vi "StandardEngineUI.vi"() -> ()   [LabVIEW 2013, in "Standard Engine Editor Node.lvclass"]
doc: "This VI is a template of the minimun components for a node UI.\nIt shows how to use the queue and the user event."
uses:
  Standard Engine Editor Node.lvclass
  <vilib>/CEF_TreeControl/Node/NodeRef.ctl
  <vilib>/CEF_TreeControl/Node/NISE_CEF_Node.lvclass
  <vilib>/NI/AMC/Message Queue.ctl
  <vilib>/NI/AMC/Message.ctl
  <vilib>/NI/Tools/Keyed Array/KeyedArray.ctl
  <vilib>/CEF_TreeControl/Node/UserEventRef.ctl
  <vilib>/CEF_TreeControl/Controls/EventCluster.ctl
  <vilib>/NI/TBM Engines/Standard Engine/Configuration/Supported Timing Sources.ctl
  Processor Assignment Mode.ctl
  <vilib>/NI/TBM Engines/Standard Engine/Configuration/Module Decimation.ctl
  <vilib>/NI/TBM Engines/Standard Engine/Configuration/Standard Engine Configuration.lvclass
  <vilib>/NI/Tag Bus Data Framework/Configuration Editor/Classes/Engine Parent/Engine Parent Editor Node.lvclass
  <vilib>/NI/TBM Engines/Standard Engine/Configuration/Standard Engine Configuration.lvclass/Standard Engine Configuration.ctl
  <vilib>/NI/TBM Engines/Standard Engine/Configuration/Module Error Configuration.ctl
  <vilib>/NI/TBM Engines/Standard Engine/Configuration/Error Actions By Category.ctl
  <vilib>/NI/Tag Bus Module Framework/runtime/error classification.ctl
  <vilib>/NI/TBM Engines/Standard Engine/Configuration/Error Actions.ctl
  <vilib>/NI/TBM Engines/Standard Engine/Configuration/Write Timing Source Type.vi
  <vilib>/NI/TBM Engines/Standard Engine/Configuration/Write Processor.vi
  <vilib>/NI/TBM Engines/Standard Engine/Configuration/Read Module Specific Configuration.vi
  <vilib>/NI/TBM Engines/Standard Engine/Configuration/Read Processor.vi
  <vilib>/NI/TBM Engines/Standard Engine/Configuration/Read Timing Source Type.vi
  <vilib>/NI/Tag Bus Data Framework/Configuration Editor/Classes/Engine Parent/Read Name.vi
  <vilib>/NI/AMC/Create Single Message.vi
  <vilib>/NI/AMC/Update Message Routing Info.vi
  <vilib>/NI/Tag Bus Module Framework/root configuration/read metadata property.vi
  <vilib>/NI/TBM Engines/Standard Engine/Configuration/Write Timing Source dt.vi
  <vilib>/NI/AMC/Send Message.vi
  <vilib>/NI/TBM Engines/Standard Engine/Configuration/Read Timing Source dt.vi
  <vilib>/NI/TBM Engines/Standard Engine/Configuration/Find Module Specific Config.vi
  <vilib>/Utility/error.llb/Error Cluster From Error Code.vi
  <vilib>/NI/Tag Bus Module Framework/root configuration/TBM configuration.lvclass
  <vilib>/NI/AMC/AMC.lvlib
  <vilib>/NI/Tag Bus Module Framework/runtime/TBM module execution interface.lvclass
  <vilib>/CEF_TreeControl/NISE_CEF_TreeControl.lvlib
  <vilib>/NI/Tools/Keyed Array/Tools_KeyedArray.lvlib
panel:
  in  "Warning Message":string="This timing source is not deterministic."
  in  "Module Decimation":T2(array[cluster]) {"Module Decimation"."Decimation" min=1}
  in  "Mode":T3
  in  "Timing Source Type":T4=enum."1 kHz Clock"
  in  "Engine Name":string
  in  "Procesor Assignment":i32 min=0
  in  "Timing Source dt":u32=5000
  in  "user event":T5
  in  "main queue":T6
  in  "node ref":T7
  # "Processor Assignment"
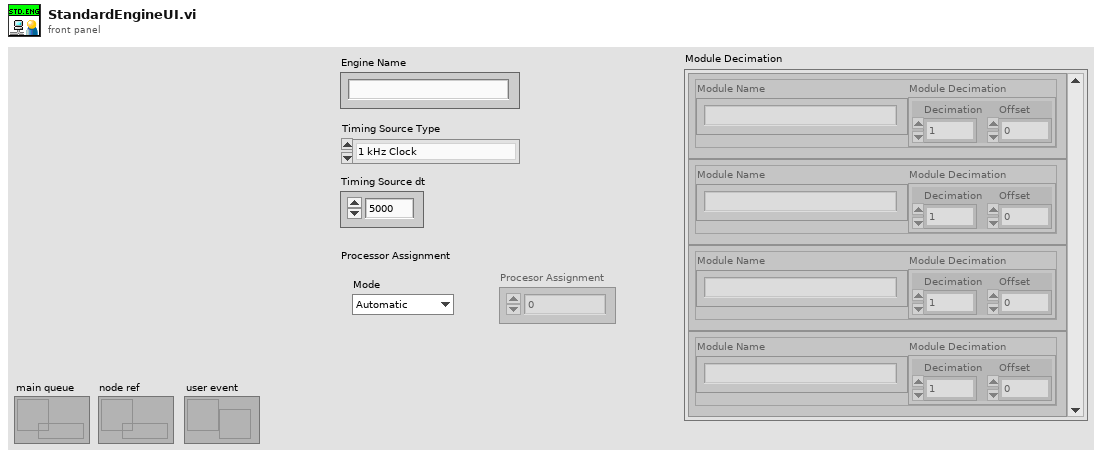
[diagram p1: front panel]
types:
  T1 = typedef "Standard Engine Configuration.lvclass/Module Decimation.ctl" = cluster{"Decimation":u16, "Offset":u16}
  T2 = cluster{"Module Name":string, "Module Decimation":T1, "Module ID":string}[]
  T3 = typedef "Standard Engine Editor Node.lvclass/Processor Assignment Mode.ctl" = enum16{"Automatic", "Manual"}
  T4 = typedef "Standard Engine Configuration.lvclass/Supported Timing Sources.ctl" = enum16{"Use Module Timing Source", "1 kHz Clock", "1 MHz Clock", "Synchronize to Scan Engine"}
  T5 = typedef "NISE_CEF_Node.lvclass/UserEventRef.ctl" = refnum<user-event>
  T6 = typedef "AMC.lvlib/Message Queue.ctl" = refnum<queue>
  T7 = typedef "NISE_CEF_Node.lvclass/NodeRef.ctl" = refnum<data-value>
  T8 = typedef "NISE_CEF_TreeControl.lvlib/EventCluster.ctl" = cluster{"command":string, "data":string}
  T9 = typedef "Standard Engine Configuration.lvclass/Module Error Configuration.ctl" = cluster{"Module Error Configuration":T10[]}
  T10 = typedef "Standard Engine Configuration.lvclass/Error Actions By Category.ctl" = cluster{"error classification":T11, "Error Actions":T12[]}
  T11 = typedef "TBM module execution interface.lvclass/error classification.ctl" = enum16{"unknown", "none", "trivial", "recoverable", "critical"}
  T12 = typedef "Standard Engine Configuration.lvclass/Error Actions.ctl" = enum16{"Clear", "Notify", "Stop Component", "Stop Engine", "Safe State", "Attempt Recovery"}
  T13 = typedef "Standard Engine Configuration.lvclass/Module Specific Configuration.ctl" = cluster{"Module ID":string, "Module Decimation":T1, "Module Error Configuration":T9}
  T14 = cluster{"Module Name":string, "Module Decimation":T1, "Module ID":string}
  T15 = enum8{"Enabled", "Disabled", "Disabled and Grayed Out"}
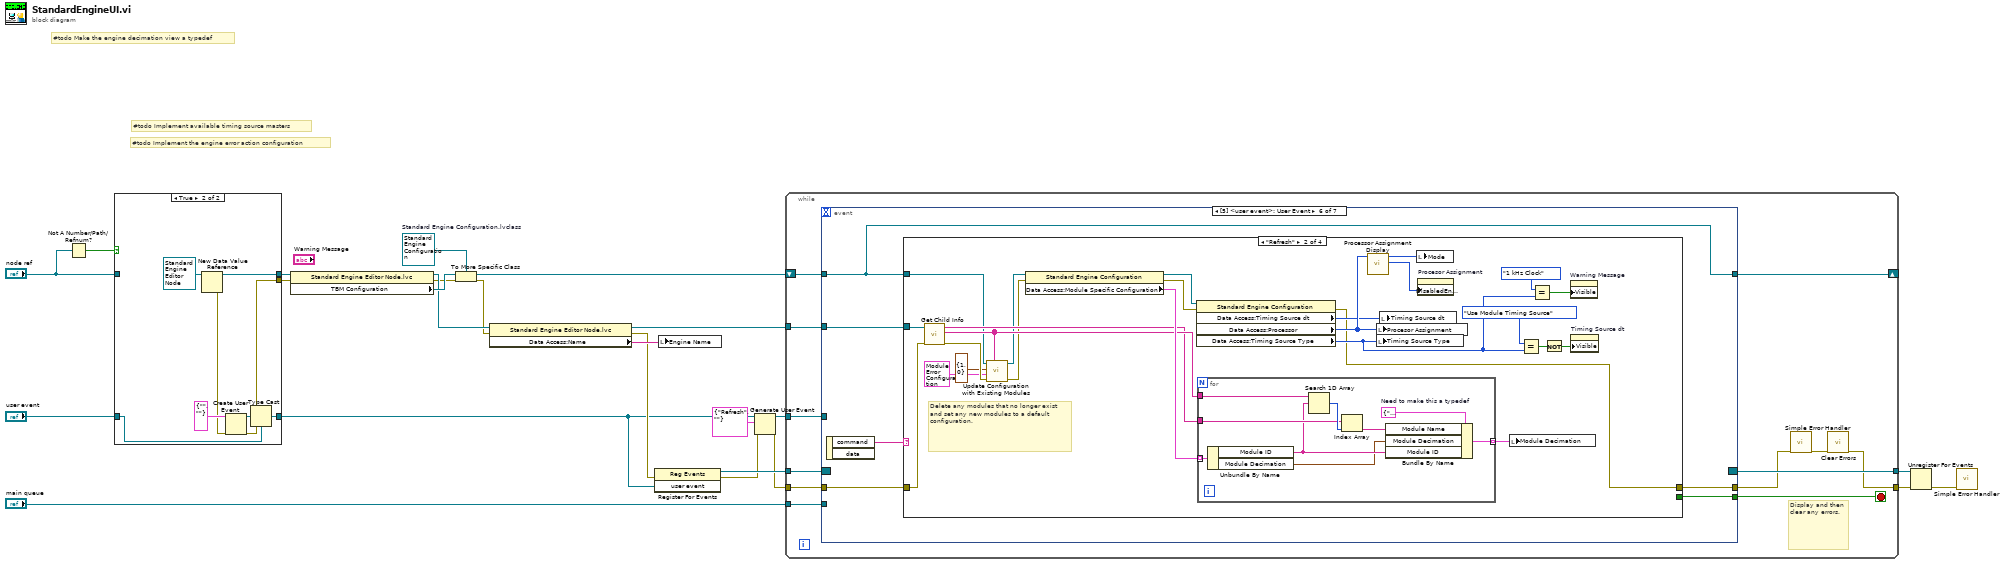
[diagram p0: block diagram]
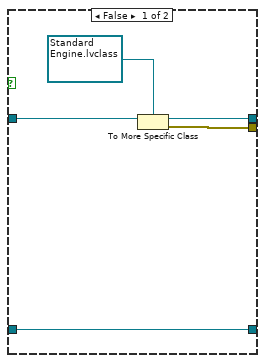
[diagram p2: hidden frame]
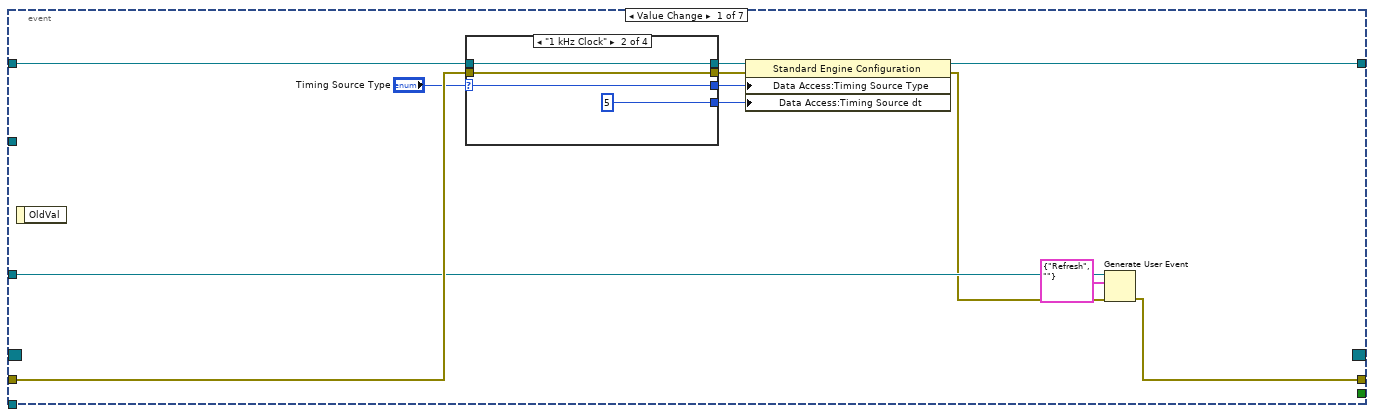
[diagram p3: hidden frame]
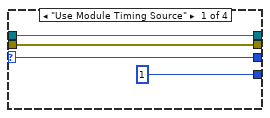
[diagram p4: hidden frame]
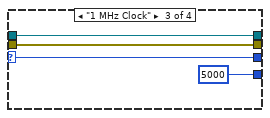
[diagram p5: hidden frame]
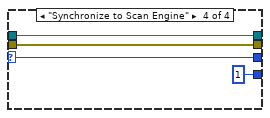
[diagram p6: hidden frame]
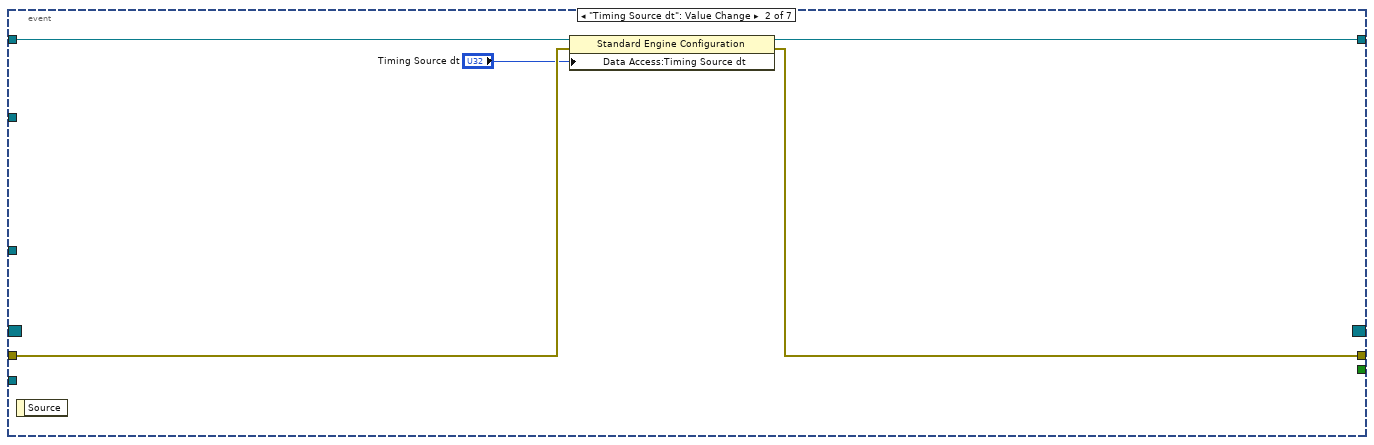
[diagram p7: hidden frame]
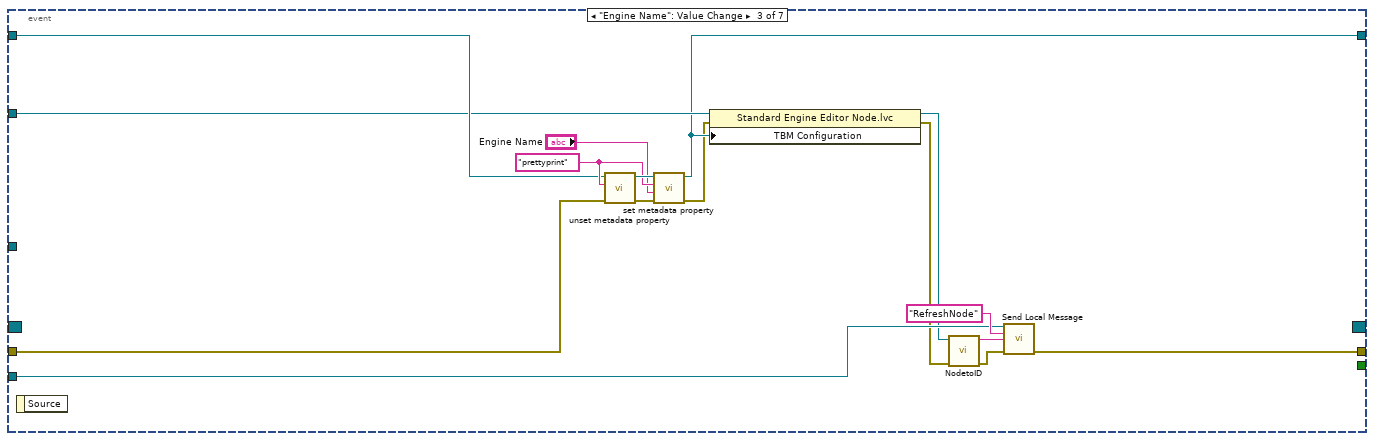
[diagram p8: hidden frame]
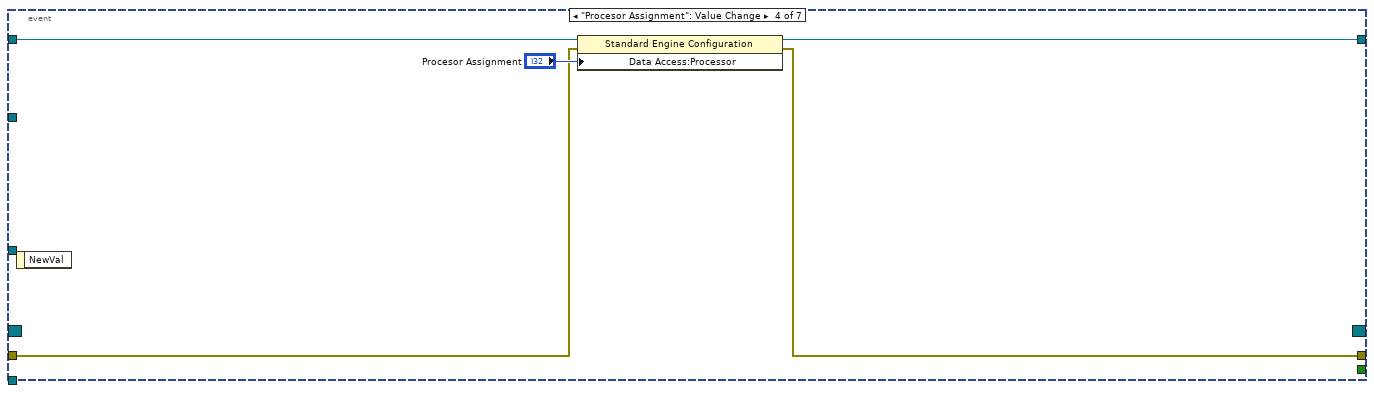
[diagram p9: hidden frame]
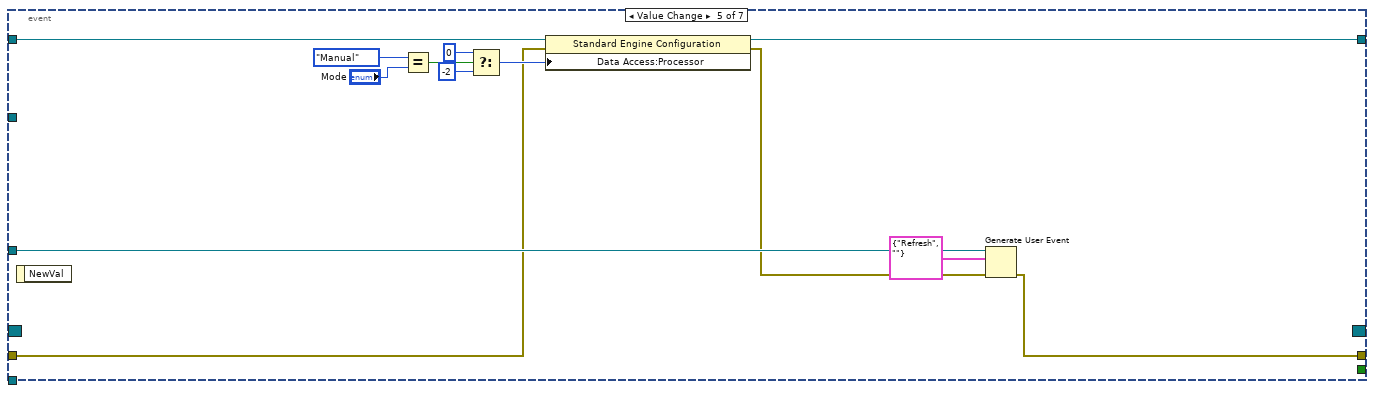
[diagram p10: hidden frame]
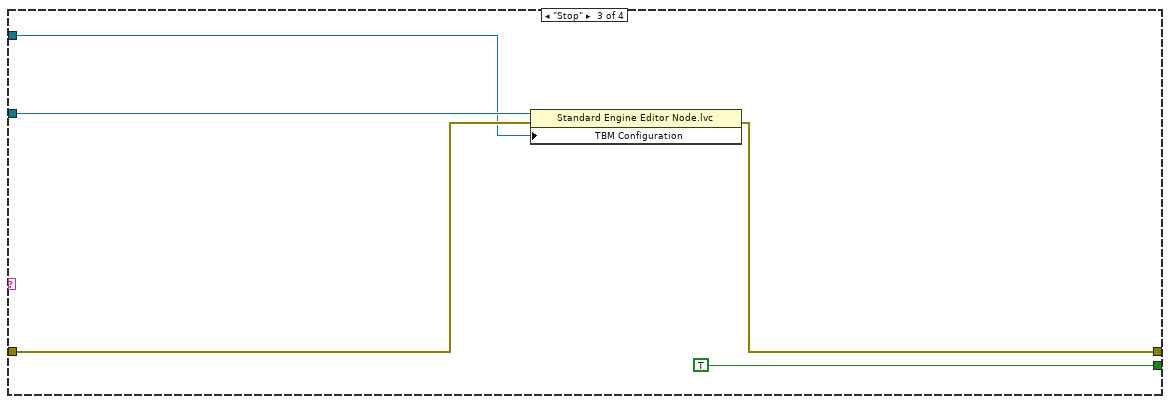
[diagram p12: hidden frame]
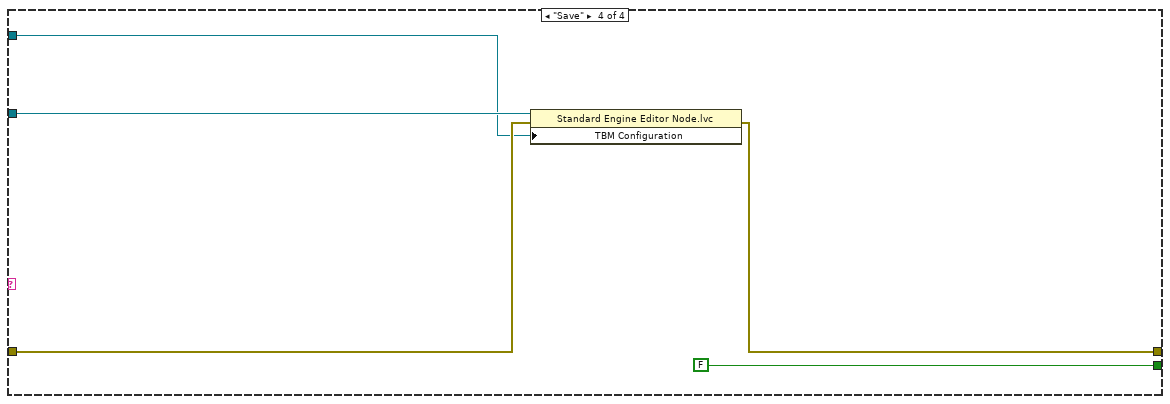
[diagram p13: hidden frame]
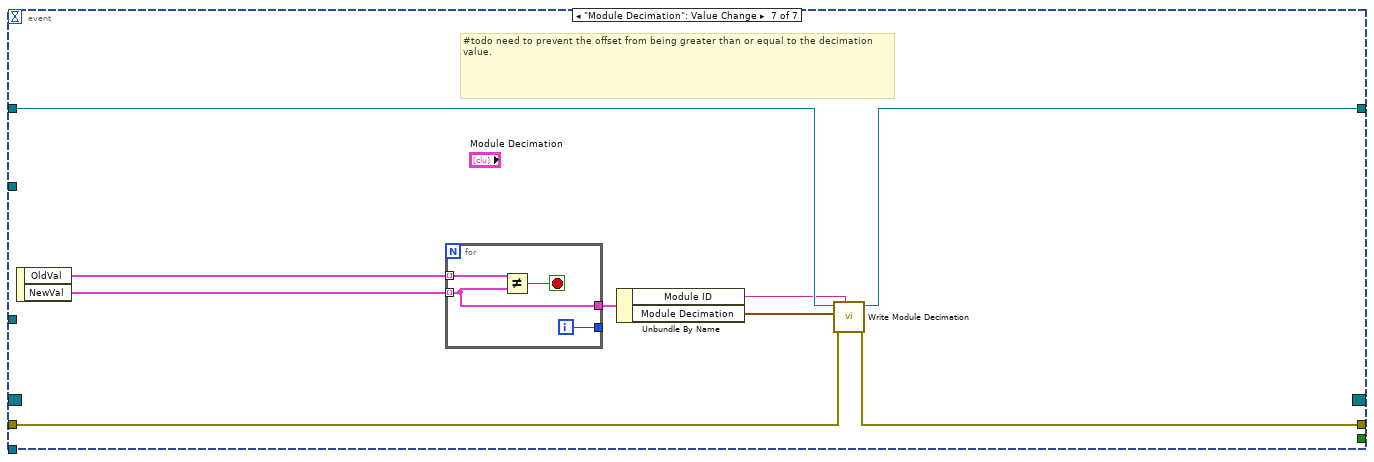
[diagram p14: hidden frame]
diagram:
  w20 = refnum<class "Standard Engine Configuration.lvclass"> refnum  # Standard Engine Configuration.lvclass
  # "#todo Implement the engine error action configuration"
  # "#todo Implement available timing source masters"
  # "#todo Make the engine decimation view a typedef"
  n1 = Not A Number/Path/Refnum?(number/path/refnum="node ref") -> (NaN/Path/Refnum?=w11:bool)
  n2 = case shown="True" w11 {
    tunnel: [w28 w32] -> w10
    tunnel: [w27 w36] -> w18
    tunnel: "node ref" -> [w26 _]
    tunnel: "user event" -> [w25 w30]
    tunnel: [w25 w31] -> w1
    frame False {
      n3 = To More Specific Class(target class=refnum<data-value> refnum ("data value reference"), reference=w26) -> (specific class reference=w27:refnum<data-value>, error out=w28:errorcluster)  [unwired: 1 in]
    }
    frame True {
      n4 = New Data Value Reference(data value=refnum<class "Standard Engine Editor Node.lvclass"> refnum ("Standard Engine Editor Node.lvclass")) -> (data value reference=w36:refnum<data-value>, error out=w33:errorcluster)  [unwired: 1 in]
      n5 = Create User Event(user event datatype=T8 {"command"="", "data"=""} ("event data"), error in=w33) -> (user event=w34:refnum<user-event>, error out=w32:errorcluster)
      n6 = Type Cast(type=w30, x=w34) -> (*(type *) &x=w31:T5)
    }
  }
  n7 = property class="Standard Engine Editor Node.lvc"(reference=w18, error in=w10) -> (reference out=w16:refnum<data-value>, error out=w15:errorcluster, "TBM Configuration"=w17:refnum<class "TBM configuration.lvclass">)
  n8 = To More Specific Class(target class=w20, reference=w17, error in=w15) -> (specific class reference=w8:refnum<class "Standard Engine Configuration.lvclass">, error out=w13:errorcluster)
  n9 = property class="Standard Engine Editor Node.lvc"(reference=w16, error in=w13) -> (reference out=w9:refnum<data-value>, error out=w7:errorcluster, "Data Access:Name"=w19:string)
  n10 = register-events(error in=w7, w1) -> (reference out=w23:refnum<event-registration>, error out=w6:errorcluster)  [unwired: 1 in]
  n11 = local write "Engine Name"(w19) -> ()
  n12 = Generate User Event(user event=w1, event data cluster=T8 {"command"="Refresh", "data"=""} ("event data"), error in=w6) -> (user event out=w3:T5, error out=w5:errorcluster)  [unwired: 1 in]
  n13 = while {
    tunnel: "main queue" -> [w49]
    tunnel: w23 -> [w48]
    tunnel: [w47] -> w22
    tunnel: [w40] -> w21
    tunnel: w5 -> [w45]
    shift-right: [w44] -> _
    shift-left: w8 -> [w39]
    tunnel: w9 -> [w43]
    tunnel: w3 -> [w38]
    stop <- w46 stop-if-true
    # "Display and then clear any errors."
    n14 = event shown="[5] <user event>: User Event" {
      selector: w48 -> [_ _ _ _ _ _ _]
      dyn-events: [_ _ _ _ _ _ _] -> w47
      timeout: _ -> [_ _ _ _ _ _ _]
      tunnel: w49 -> [_ _ w97 _ _ _ _]
      tunnel: [_ _ _ _ _ w122 _] -> w46
      tunnel: [w51 w79 w95 w99 w105 w119 w170] -> w42
      tunnel: w45 -> [w58 w80 w90 w100 w104 w120 w171]
      tunnel: w39 -> [w60 w82 w89 w103 w116 w117 w174]
      tunnel: [w61 w81 w86 w102 w115 w117 w173] -> w44
      tunnel: w43 -> [_ _ w87 _ _ w121 _]
      tunnel: w38 -> [w53 _ _ _ w107 _ _]
      event Value Change {
        n15 = event-data() -> ()  [unwired: 1 in, 1 out]
        n16 = case shown="\"1 kHz Clock\"" "Timing Source Type" {
          selector: "Timing Source Type" -> [w65 w69 w71 w75]
          tunnel: w60 -> [w64 w68 w73 w77]
          tunnel: [w64 w68 w73 w77] -> w59
          tunnel: w58 -> [w63 w67 w72 w76]
          tunnel: [w63 w67 w72 w76] -> w57
          tunnel: [w65 w69 w71 w75] -> w50
          tunnel: [u32 1 ("Timing Source dt") u32 5 ("Timing Source dt") u32 5000 ("Timing Source dt") u32 1 ("Timing Source dt")] -> w55
          frame "Use Module Timing Source" {
          }
          frame "1 kHz Clock" {
          }
          frame "1 MHz Clock" {
          }
          frame "Synchronize to Scan Engine" {
          }
        }
        n17 = property class="Standard Engine Configuration"(reference=w59, error in=w57, "Data Access:Timing Source Type"=w50, "Data Access:Timing Source dt"=w55) -> (reference out=w61:refnum<class "Standard Engine Configuration.lvclass">, error out=w52:errorcluster)
        n18 = Generate User Event(user event=w53, event data cluster=T8 {"command"="Refresh", "data"=""} ("event data"), error in=w52) -> (error out=w51:errorcluster)  [unwired: 1 in, 1 out]
      }
      event "Timing Source dt": Value Change {
        n19 = event-data() -> ()  [unwired: 1 in, 1 out]
        n20 = property class="Standard Engine Configuration"(reference=w82, error in=w80, "Data Access:Timing Source dt"="Timing Source dt") -> (reference out=w81:refnum<class "Standard Engine Configuration.lvclass">, error out=w79:errorcluster)
      }
      event "Engine Name": Value Change {
        w91 = "prettyprint" ("key")
        n21 = event-data() -> ()  [unwired: 1 in, 1 out]
        n22 = call <vilib>:"unset metadata property.vi"("error in"=w90, "key"=w91, "configuration in"=w89) -> ("error out"=w92:errorcluster, "configuration out"=w93:refnum<class "Standard Engine Configuration.lvclass">)  [unwired: 7 in]
        n23 = call <vilib>:"set metadata property.vi"("error in"=w92, "value"="Engine Name", "key"=w91, "configuration in"=w93) -> ("error out"=w85:errorcluster, "configuration out"=w86:refnum<class "Standard Engine Configuration.lvclass">)  [unwired: 6 in]
        n24 = property class="Standard Engine Editor Node.lvc"(reference=w87, error in=w85, "TBM Configuration"=w86) -> (reference out=w83:refnum<data-value>, error out=w84:errorcluster)
        n25 = call <vilib>:"NodetoID.vi"("error in"=w84, "node ref"=w83) -> ("error out"=w94:errorcluster, "ID"=w96:string)  [unwired: 8 in]
        n26 = call <vilib>:"Send Local Message.vi"("message queue in"=w97, "message name"="RefreshNode" ("Message Name"), "message value"=w96, "error in"=w94) -> ("error out"=w95:errorcluster)  [unwired: 9 in, 2 out]
      }
      event "Procesor Assignment": Value Change {
        n27 = event-data() -> ()  [unwired: 1 in, 1 out]
        n28 = property class="Standard Engine Configuration"(reference=w103, error in=w100, "Data Access:Processor"="Procesor Assignment") -> (reference out=w102:refnum<class "Standard Engine Configuration.lvclass">, error out=w99:errorcluster)
      }
      event Value Change {
        n29 = event-data() -> ()  [unwired: 1 in, 1 out]
        n30 = Equal?(x=Processor_Assignment_Mode."Manual", y="Mode") -> (x = y?=w109:bool)
        n31 = Select(t=0, s=w109, f=-2 ("Processor")) -> (s? t:f=w110:i32)
        n32 = property class="Standard Engine Configuration"(reference=w116, error in=w104, "Data Access:Processor"=w110) -> (reference out=w115:refnum<class "Standard Engine Configuration.lvclass">, error out=w106:errorcluster)
        n33 = Generate User Event(user event=w107, event data cluster=T8 {"command"="Refresh", "data"=""} ("event data"), error in=w106) -> (error out=w105:errorcluster)  [unwired: 1 in, 1 out]
      }
      event User Event {
        n34 = event-data() -> ("command"=w118:string)  [unwired: 1 in, 1 out]
        n35 = case shown="\"Refresh\"" w118 {
          tunnel: [_ _ TRUE FALSE] -> w122
          tunnel: w121 -> [_ w143 w161 w166]
          tunnel: w120 -> [w123 w140 w160 w165]
          tunnel: [w123 w129 w159 w164] -> w119
          tunnel: w117 -> [_ w128 w158 w163]
          frame Default {
          }
          frame "Refresh" {
            # "Delete any modules that no longer exist and set any new modules to a default configuration."
            n36 = call "Get Child Info.vi"("error in (no error)"=w140, "Data Value Reference in"=w143) -> ("error out"=w146:errorcluster, "Instance Identifier"=w142:string[], "Display Names"=w141:string[])  [unwired: 7 in]
            n37 = call <vilib>:"Update Configuration with Existing Modules.vi"("Module IDs"=w142, "error in"=w146, "Default Module Error Configuration"=T9 {"Module Error Configuration"=[{"error classification"=enum."unknown", "Error Actions"=[enum."Stop Engine"]}, {"error classification"=enum."none", "Error Actions"=[enum."Stop Engine"]}, {"error classification"=enum."trivial", "Error Actions"=[enum."Stop Engine"]}, {"error classification"=enum."recoverable", "Error Actions"=[enum."Stop Engine"]}, {"error classification"=enum."critical", "Error Actions"=[enum."Stop Engine"]}]} ("Module Error Configuration"), "Default Module Decimation"=T1 {"Decimation"=1, "Offset"=0}, "Standard Engine Configuration in"=w128) -> ("error out"=w125:errorcluster, "Standard Engine Configuration out"=w127:refnum<class "Standard Engine Configuration.lvclass">)  [unwired: 5 in]
            n38 = property class="Standard Engine Configuration"(reference=w127, error in=w125) -> (reference out=w126:refnum<class "Standard Engine Configuration.lvclass">, error out=w124:errorcluster, "Data Access:Module Specific Configuration"=w147:T13[])
            n39 = property class="Standard Engine Configuration"(reference=w126, error in=w124) -> (error out=w129:errorcluster, "Data Access:Timing Source dt"=w130:u32, "Data Access:Processor"=w131:i32, "Data Access:Timing Source Type"=w136:T4)  [unwired: 1 out]
            n40 = for {
              tunnel: w147 -> [w157] mode=indexing
              tunnel: w142 -> [w156]
              tunnel: w141 -> [w154]
              tunnel: [w149] -> w148 mode=indexing
              w153 = T14 {"Module Name"="", "Module Decimation"={"Decimation"=1, "Offset"=0}, "Module ID"=""}  # Need to make this a typedef
              n41 = Unbundle By Name(w157) -> ("Module ID"=w151:string, "Module Decimation"=w150:T1)
              n42 = Search 1D Array(1D array=w156, element=w151) -> (index of element=w155:i32)  [unwired: 1 in]
              n43 = Index Array(array=w154, index=w155) -> (element=w152:string)
              n44 = Bundle By Name(cluster=w153, "Module Name"=w152, "Module Decimation"=w150, "Module ID"=w151) -> (w149:T14)
            }
            n45 = call "Processor Assignment Display.vi"("Data Access:Processor"=w131) -> ("Enabled?"=w133:T15, "Mode"=w132:T3)  [unwired: 9 in]
            n46 = local write "Procesor Assignment"(w131) -> ()
            n47 = local write "Timing Source Type"(w136) -> ()
            n48 = local write "Timing Source dt"(w130) -> ()
            n49 = local write "Mode"(w132) -> ()
            n50 = property on="Procesor Assignment" class="DigNum (strict)"("DisabledEnum"=w133) -> ()  [unwired: 2 in, 2 out]
            n51 = local write "Module Decimation"(w148) -> ()
            n52 = Equal?(x=Supported_Timing_Sources."Use Module Timing Source" ("Timing Source Type"), y=w136) -> (x = y?=w138:bool)
            n53 = Equal?(x=Supported_Timing_Sources."1 kHz Clock" ("Timing Source Type"), y=w136) -> (x = y?=w134:bool)
            n54 = Not(x=w138) -> (.not. x?=w139:bool)
            n55 = property on="Warning Message" class="Str"("Visible"=w134) -> ()  [unwired: 2 in, 2 out]
            n56 = property on="Timing Source dt" class="DigNum (strict)"("Visible"=w139) -> ()  [unwired: 2 in, 2 out]
          }
          frame "Stop" {
            n57 = property class="Standard Engine Editor Node.lvc"(reference=w161, error in=w160, "TBM Configuration"=w158) -> (error out=w159:errorcluster)  [unwired: 1 out]
          }
          frame "Save" {
            n58 = property class="Standard Engine Editor Node.lvc"(reference=w166, error in=w165, "TBM Configuration"=w163) -> (error out=w164:errorcluster)  [unwired: 1 out]
          }
        }
      }
      event "Module Decimation": Value Change {
        # "#todo need to prevent the offset from being greater than or equal to the decimation value."
        n59 = event-data() -> ("OldVal"=w176:T2, "NewVal"=w175:T2)  [unwired: 1 in]
        n60 = for {
          tunnel: w176 -> [w180] mode=indexing
          tunnel: w175 -> [w177] mode=indexing
          tunnel: [w178] -> _
          tunnel: [w177] -> w169
          i -> [w178]
          stop <- w179 stop-if-true
          n61 = Not Equal?(x=w180, y=w177) -> (x != y?=w179:bool)
        }
        n62 = Unbundle By Name(w169) -> ("Module ID"=w168:string, "Module Decimation"=w172:T1)
        n63 = call <vilib>:"Write Module Decimation.vi"("Module ID"=w168, "error in"=w171, "Module Decimation"=w172, "Standard Engine Repo Data in"=w174) -> ("error out"=w170:errorcluster, "Standard Engine Repo Data out"=w173:refnum<class "Standard Engine Configuration.lvclass">)  [unwired: 6 in]
      }
    }
    n64 = call <vilib>:"Simple Error Handler.vi"("error in (no error)"=w42) -> ("error out"=w41:errorcluster)  [unwired: 4 in, 4 out]
    n65 = call <vilib>:"Clear Errors.vi"("error in (no error)"=w41) -> ("error out"=w40:errorcluster)  [unwired: 6 in]
  }
  n66 = Unregister For Events(event registration refnum=w22, error in=w21) -> (error out=w14:errorcluster)
  n67 = call <vilib>:"Simple Error Handler.vi"("error in (no error)"=w14) -> ()  [unwired: 4 in, 5 out]
